vi "Vr_Wr2.vi"(7 "Phirp":dbl[](array[numeric]), 9 "Phir":dbl[](array[numeric]), 10 "Ydrp":dbl[](array[numeric]), 11 "Xdrp":dbl[](array[numeric])) -> (3 "VLW":T1)   [LabVIEW 2011]
uses:
  <vilib>/Analysis/Matrix/Datatypes/RealMatrix.ctl
  <vilib>/Analysis/Matrix/Numeric/Conversions/Array To Matrix - RA.vi
  <vilib>/Analysis/_algsub.llb/Real PseudoInverse Matrix.vi
  <vilib>/Analysis/Matrix/NI_Matrix.lvlib
  <vilib>/Analysis/NI_AALPro.lvlib
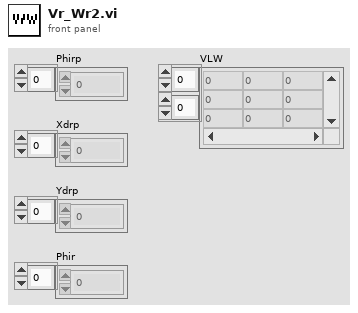
[diagram p1: front panel]
types:
  T1 = typedef "NI_Matrix.lvlib/RealMatrix.ctl" = dbl[][]
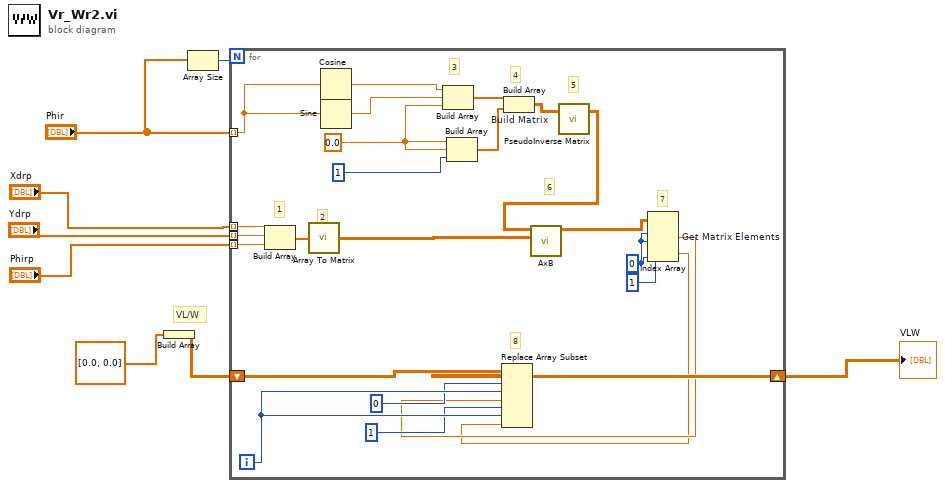
[diagram p0: block diagram]
diagram:
  # "VL/W"
  n1 = Build Array(dbl[] [0.0, 0.0]) -> (w7:T1)
  n2 = Array Size(array="Phir") -> (size(s)=w5:i32)
  n3 = for {
    N: w5 -> [_]
    tunnel: "Phir" -> [w32] mode=indexing
    tunnel: "Xdrp" -> [w23] mode=indexing
    tunnel: "Ydrp" -> [w24] mode=indexing
    tunnel: "Phirp" -> [w25] mode=indexing
    shift-right: [w14] -> w8
    shift-left: w7 -> [w15]
    i -> [w13]
    w17 = 0 ("index (col)")
    w28 = 0.0
    # "6"
    # "2"
    # "8"
    # "7"
    # "5"
    # "4"
    # "3"
    # "1"
    n4 = Build Array(w23, w24, w25) -> (w22:dbl[])
    n5 = call-poly <vilib>:"Array To Matrix.vi"("Real 1D Array"=w22) -> ("Real Matrix (Column Vector)"=w21:T1)
    n6 = Cosine(x=w32) -> (cos(x)=w30:dbl)
    n7 = Sine(x=w32) -> (sin(x)=w31:dbl)
    n8 = Build Array(w30, w31, w28) -> (w27:dbl[])
    n9 = Build Array(w28, w28, 1) -> (w26:dbl[])
    n10 = Build Array "Build Matrix"(w27, w26) -> (w20:T1)
    n11 = call-poly <vilib>:"PseudoInverse Matrix.vi"("Input Matrix"=w20) -> ("PseudoInverse Matrix"=w19:T1)  [unwired: 1 in, 1 out]
    n12 = call "AxB.vi"("B"=w21, "A"=w19) -> ("AxB"=w16:T1)  [unwired: 9 in]
    n13 = Index Array "Get Matrix Elements"(array=w16, index (row) #1=w17, index (col) #1=w17, index (row) #2=1 ("index (row)"), index (col) #2=w17) -> (element #1=w10:dbl, element #2=w9:dbl)
    n14 = Replace Array Subset(array=w15, new element #1=w10, index (row) #1=0 ("disabled index (row)"), index (col) #1=w13, new element #2=w9, index (row) #2=1 ("disabled index (row)"), index (col) #2=w13) -> (w14:T1)
  }
  "VLW" <- w8
